vi "UI Message Loop_Start_InitializeFP.vi"(11 "C&C Data in":T1={"Hardware Configuration"={"COM Port"="", "Reference Distance"=0.0, "Sensor SN"=""}, "Logging Configuration"={"Log File Base Path"=path "", "Datafile Ref"=refnum, "Database Ref"=refnum}, "UI Refs"={"Start Ref"=refnum, "Settings Ref"=refnum, "Stop Ref"=refnum, "Exit Ref"=refnum, "Status Ref"=refnum, "Data Ref"=refnum, "StatusBox Ref"=refnum, "Location Ref"=refnum, "Operator Ref"=refnum, "Time Ref"=refnum, "Test in Progess Ref"=refnum}, "Calibration Data"={"calibrationID"=0, "operatorID"=0, "sensorID"=0, "start_time"="", "end_time"="", "offset"=0.0, "offset_units"="", "ring_time"=0.0, "error"=0.0, "Passed"=0, "data_storage_location"="", "comments"=""}, "Time Elapsed"=0, "Samples Required"=480} {"Hardware Configuration"."Reference Distance" format="%.3g"}) -> (3 "C&C Data out":T1={"Hardware Configuration"={"COM Port"="", "Reference Distance"=0.0, "Sensor SN"=""}, "Logging Configuration"={"Log File Base Path"=path "", "Datafile Ref"=refnum, "Database Ref"=refnum}, "UI Refs"={"Start Ref"=refnum, "Settings Ref"=refnum, "Stop Ref"=refnum, "Exit Ref"=refnum, "Status Ref"=refnum, "Data Ref"=refnum, "StatusBox Ref"=refnum, "Location Ref"=refnum, "Operator Ref"=refnum, "Time Ref"=refnum, "Test in Progess Ref"=refnum}, "Calibration Data"={"calibrationID"=0, "operatorID"=0, "sensorID"=0, "start_time"="", "end_time"="", "offset"=0.0, "offset_units"="", "ring_time"=0.0, "error"=0.0, "Passed"=0, "data_storage_location"="", "comments"=""}, "Time Elapsed"=0, "Samples Required"=480} {"Hardware Configuration"."Reference Distance" format="%.3g"})   [LabVIEW 2018]
uses:
  Settings/Settings.ctl
  Acquisition/Hardware Configuration.ctl
  Logging/Logging Configuration.ctl
  <vilib>/addons/database/Connection.llb/Conn ObjectReference.ctl
  Controls/Location Ring.ctl
  Controls/Time Remaining.ctl
  Acquisition/Acquisition.lvlib
  <vilib>/addons/database/NI_Database_API.lvlib
  Logging/Logging.lvlib
  Settings/Settings.lvlib
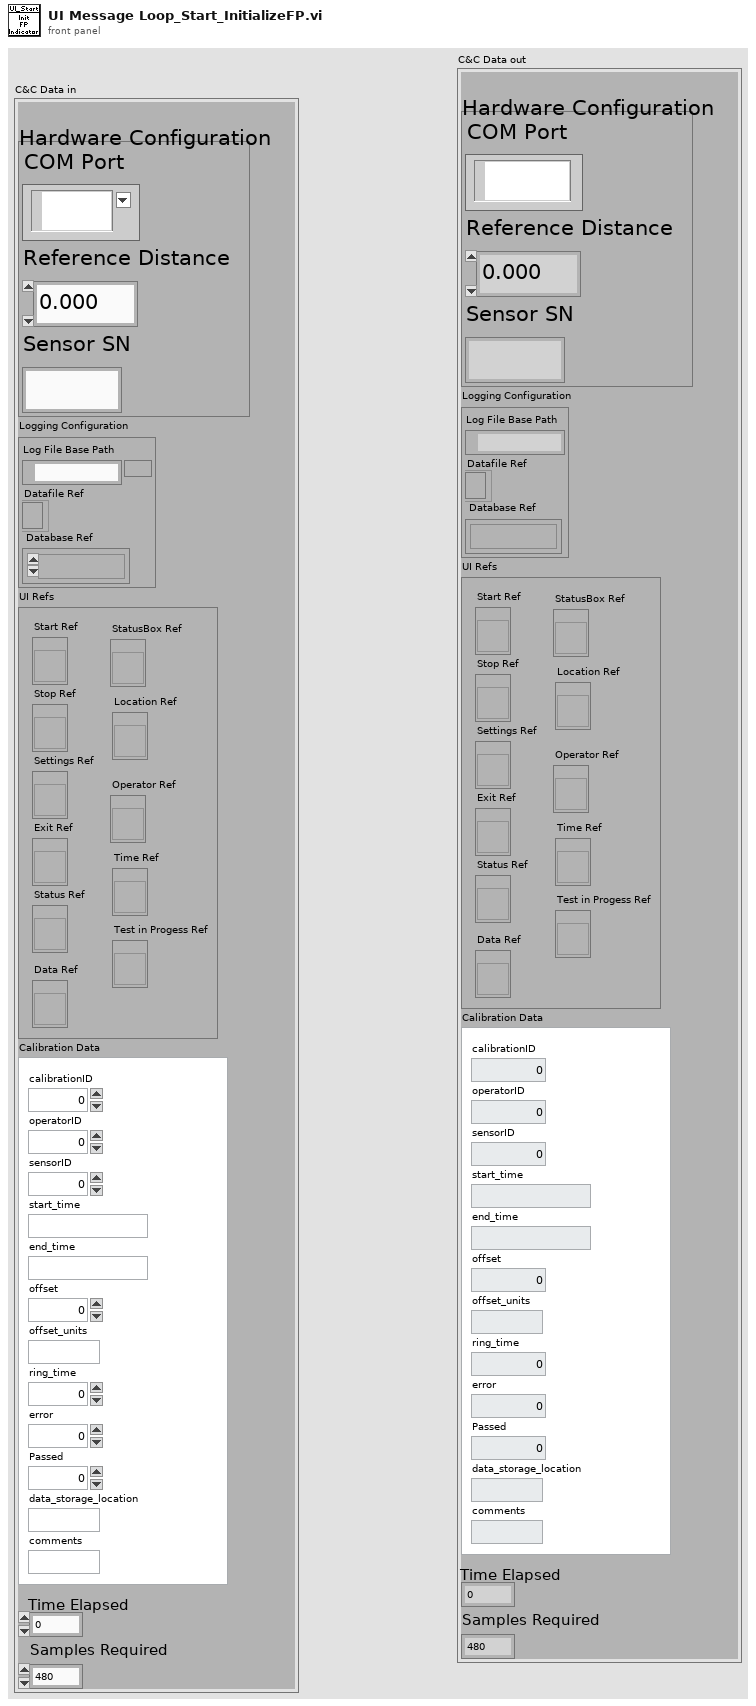
[diagram p1: front panel]
types:
  T1 = typedef "Settings.lvlib/Settings.ctl" = cluster{"Hardware Configuration":T2, "Logging Configuration":T3, "UI Refs":cluster{"Start Ref":refnum<vi>, "Settings Ref":refnum<vi>, "Stop Ref":refnum<vi>, "Exit Ref":refnum<vi>, "Status Ref":refnum<vi>, "Data Ref":refnum<vi>, "StatusBox Ref":refnum<vi>, "Location Ref":refnum<vi>, "Operator Ref":refnum<vi>, "Time Ref":refnum<vi>, "Test in Progess Ref":refnum<vi>}, "Calibration Data":cluster{"calibrationID":u16, "operatorID":u16, "sensorID":u16, "start_time":string, "end_time":string, "offset":dbl, "offset_units":string, "ring_time":dbl, "error":dbl, "Passed":u8, "data_storage_location":string, "comments":string}, "Time Elapsed":u16, "Samples Required":u16}
  T2 = typedef "Acquisition.lvlib/Hardware Configuration.ctl" = cluster{"COM Port":refnum<visa-resource-name>, "Reference Distance":dbl, "Sensor SN":string}
  T3 = typedef "Logging.lvlib/Logging Configuration.ctl" = cluster{"Log File Base Path":path, "Datafile Ref":refnum<file>, "Database Ref":T4}
  T4 = typedef "NI_Database_API.lvlib/Conn ObjectReference.ctl" = refnum<k1>
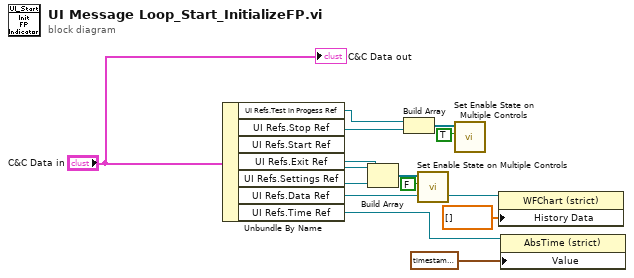
[diagram p0: block diagram]
diagram:
  n1 = Unbundle By Name("C&C Data in") -> ("UI Refs.Test in Progess Ref"=w13:refnum<vi>, "UI Refs.Stop Ref"=w6:refnum<vi>, "UI Refs.Start Ref"=w7:refnum<vi>, "UI Refs.Exit Ref"=w8:refnum<vi>, "UI Refs.Settings Ref"=w9:refnum<vi>, "UI Refs.Data Ref"=w11:refnum<vi>, "UI Refs.Time Ref"=w12:refnum<vi>)
  n2 = Build Array(w7, w8, w9) -> (w3:refnum<vi>[])
  n3 = Build Array(w13, w6) -> (w4:refnum<vi>[])
  n4 = call "Set Enable State on Multiple Controls.vi"("Enable?"=FALSE, "Controls"=w3) -> ()  [unwired: 10 in]
  n5 = call "Set Enable State on Multiple Controls.vi"("Enable?"=TRUE, "Controls"=w4) -> ()  [unwired: 10 in]
  n6 = property class="WFChart (strict)"(reference=w11, "History Data"=dbl[] []) -> ()  [unwired: 1 in, 2 out]
  n7 = property class="AbsTime (strict)"(reference=w12, "Value"=timestamp(-68400 s since 1904-01-01) ("Time Stamp")) -> ()  [unwired: 1 in, 2 out]
  "C&C Data out" <- "C&C Data in"
